vi "Encode UTF-8 String.vi"(5 "Prepend BOM (F)":bool, 7 "Output Encoding (UTF-16LE)":T1=enum."UTF-16LE", 9 "error in (no error)":errorcluster, 10 "UTF-8 String":refnum<class "UTF-8 String.lvclass">) -> (1 "error out":errorcluster, 2 "Encoded String":string)   [LabVIEW 2020, in "G-Unicode.lvlib" / "UTF-8 String.lvclass"]
doc: "Encodes the input <b>UTF-8 String</b> using the specified <b>Output Encoding</b>."
uses:
  UTF-8 String.lvclass
  G-Unicode.lvlib
  Unicode/Controls/String Encoding.ctl
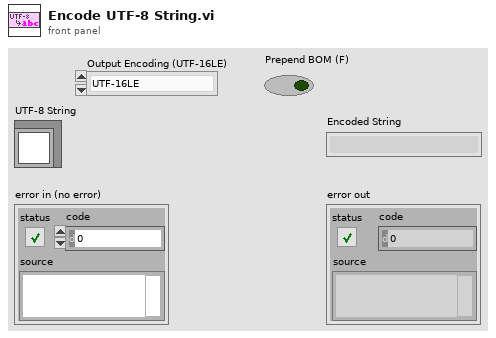
[diagram p1: front panel]
types:
  T1 = typedef "G-Unicode.lvlib/String Encoding.ctl" = enum16{"ANSI", "UTF-8", "UTF-16LE", "UTF-16BE", "Unknown"}
  T2 = typedef "G-Unicode.lvlib/Encoded UTF-8 String.ctl" = string
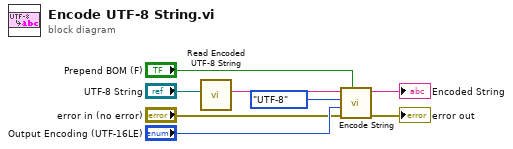
[diagram p0: block diagram]
diagram:
  n1 = call "Read Encoded UTF-8 String.vi"("UTF-8 String"="UTF-8 String") -> ("Encoded UTF-8 String"=w7:T2)  [unwired: 10 in]
  n2 = call "Encode String.vi"("Prepend BOM (F)"="Prepend BOM (F)", "error in"="error in (no error)", "Output Encoding (UTF-16LE)"="Output Encoding (UTF-16LE)", "Input Encoding (ANSI)"=String_Encoding."UTF-8", "String in"=w7) -> ("error out"=→"error out":errorcluster, "String out"=→"Encoded String":string)  [unwired: 5 in]
